vi "Lift Scale Potentiometer.vi"(0 "Potentiometer In":dbl, 5 "Limit Switches":T5, 7 "Initial Upper Value":dbl=1.0, 9 "Initial Lower Value":dbl=0.44, 11 "From Shift":dbl, 12 "Upper Limit Index ( 0 - 3 )":i32, 13 "Lower Limit Index (0 - 3 )":i32=1) -> (4 "Scaled Value Out":dbl, 15 "To Shift":dbl)   [LabVIEW 2014]
uses:
  <vilib>/Rock Robotics/WPI/Switch/WPI_SwitchDevRef.ctl
  <vilib>/Rock Robotics/SystemInterfaces/DIO/FPGA_DIOChannel.ctl
  <vilib>/Rock Robotics/SystemInterfaces/Typedef/FPGA_TypedefDigitalModule.ctl
  <vilib>/Rock Robotics/SystemInterfaces/Counter/FPGA_CounterCtrSystemIndex.ctl
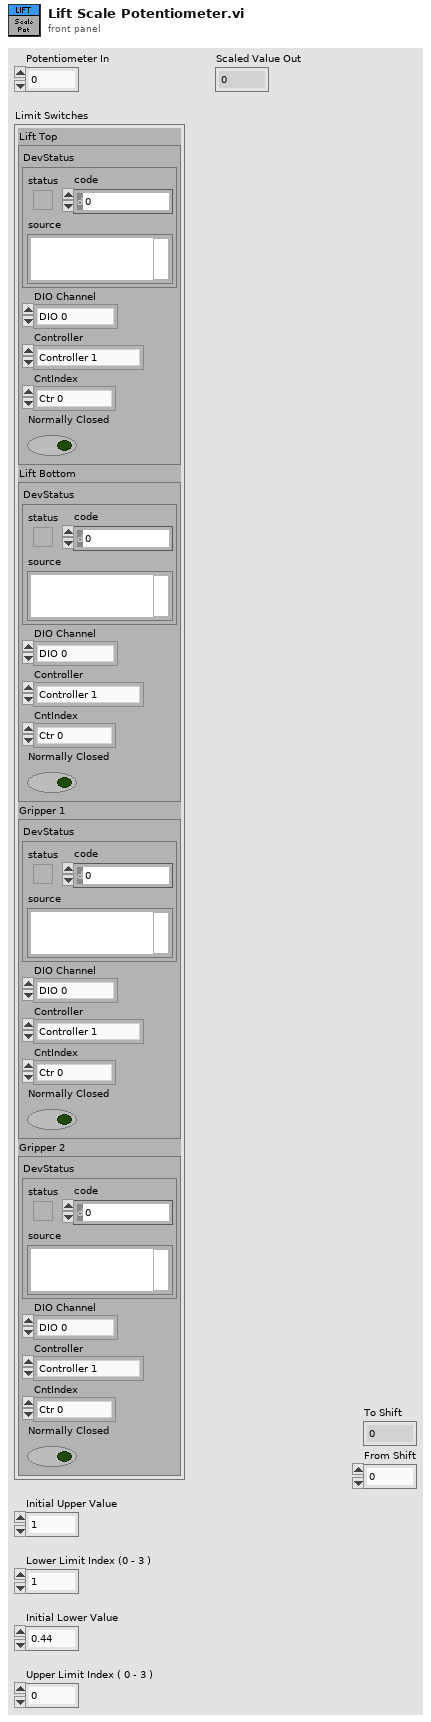
[diagram p1: front panel]
types:
  T1 = typedef "WPI_SwitchDevRef.ctl" = cluster{"DevStatus":errorcluster, "DIO Channel":T2, "Controller":T3, "CntIndex":T4, "Normally Closed":bool}
  T2 = typedef "FPGA_DIOChannel.ctl" = enum8{"DIO 0", "DIO 1", "DIO 2", "DIO 3", "DIO 4", "DIO 5", "DIO 6", "DIO 7", "DIO 8", "DIO 9", "DIO MXP 0", "DIO MXP 1", "DIO MXP 2", "DIO MXP 3", "DIO MXP 4", "DIO MXP 5", "DIO MXP 6", "DIO MXP 7", "DIO MXP 8", "DIO MXP 9", "DIO MXP 10", "DIO MXP 11", "DIO MXP 12", "DIO MXP 13", "DIO MXP 14", "DIO MXP 15", "Invalid"}
  T3 = typedef "FPGA_TypedefDigitalModule.ctl" = enum16{"Controller 1"}
  T4 = typedef "FPGA_CounterCtrSystemIndex.ctl" = enum8{"Ctr 0", "Ctr 1", "Ctr 2", "Ctr 3", "Ctr 4", "Ctr 5", "Ctr 6", "Ctr 7", "Invalid"}
  T5 = cluster{"Lift Top":T1, "Lift Bottom":T1, "Gripper 1":T1, "Gripper 2":T1}
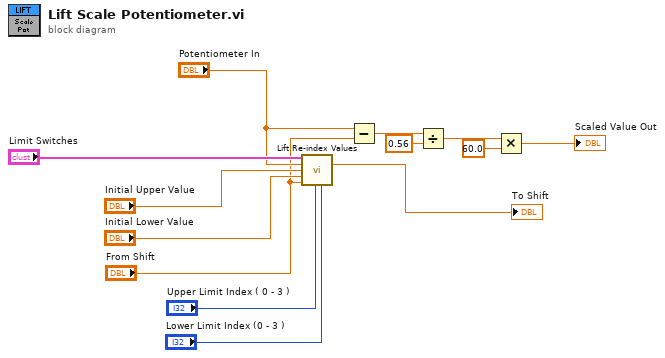
[diagram p0: block diagram]
diagram:
  n1 = call "Lift Re-index Values.vi"("Limit Switches"="Limit Switches", "Input for Re-indexing"="Potentiometer In", "Initial Upper Value"="Initial Upper Value", "Initial Lower Value"="Initial Lower Value", "Current Lower Value"="From Shift", "Upper Limit Index ( 0 - 3 )"="Upper Limit Index ( 0 - 3 )", "Lower Limit Index ( 0 - 3 )"="Lower Limit Index (0 - 3 )") -> ("Re-indexed Value"=→"To Shift":dbl)  [unwired: 8 in]
  n2 = Subtract(x="Potentiometer In", y="From Shift") -> (x-y=w6:dbl)
  n3 = Divide(x=w6, y=0.56) -> (x/y=w10:dbl)
  n4 = Multiply(x=w10, y=60.0) -> (x*y=→"Scaled Value Out":dbl)
